vi "changeMode.vi"(8 "error in (no error)":errorcluster, 9 "Mode":T1, 10 "ElectrometerController in":refnum<class "ElectrometerController.lvclass">, 11 "ReadyState in":refnum<class "ReadyState.lvclass">) -> (0 "error out":errorcluster, 2 "ElectrometerController out":refnum<class "ElectrometerController.lvclass">, 3 "ReadyState out":refnum<class "ReadyState.lvclass">)   [LabVIEW 2016, in "ReadyState.lvclass"]
uses:
  ReadyState.lvclass
  ElectrometerController/ElectrometerController.lvclass
  Modes.ctl
  ts_electrometeruserevents/Typedefs/StateValue.ctl
  ts_electrometeruserevents/Typedefs/CommandValue.ctl
  ts_electrometeruserevents/Typedefs/PubDataSV.ctl
  ts_sallv_calibrationelectrometer/DataTypes/logevent_measureType.ctl
  ElectrometerController/ElectrometerController.lvclass/ElectrometerController.ctl
  ts_electrometeruserevents/PubSubDataEvent/PubSubDataEvent.lvclass
  Electrometer.lvclass
  ElectrometerConfiguration/ElectrometerInternalConfiguration.lvclass
  ts_electrometeruserevents/Typedefs/ElectrometerTypedefs.lvlib
  ts_sallv_calibrationelectrometer/SALLV_calibrationElectrometer.lvlib
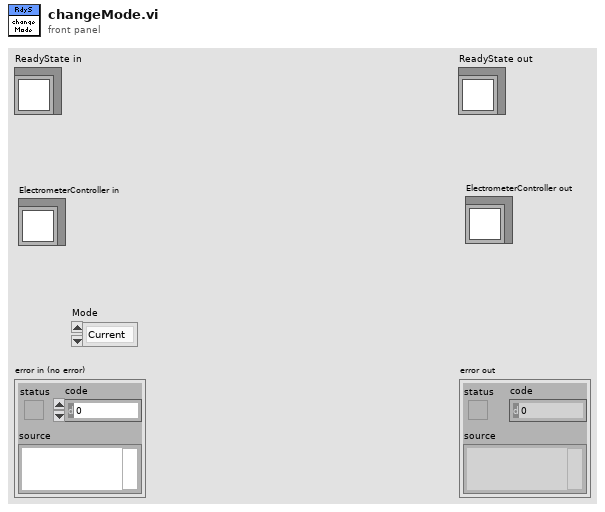
[diagram p1: front panel]
types:
  T1 = typedef "Electrometer.lvclass/Modes.ctl" = enum16{"Current", "Charge"}
  T2 = typedef "SALLV_calibrationElectrometer.lvlib/logevent_measureType.ctl" = cluster{"electId":i16, "mode":u16, "priority":i32}
  T3 = typedef "ElectrometerTypedefs.lvlib/PubDataSV.ctl" = enum16{"DetailedState", "ErrorCode", "Heartbeat", "LoopTime_ms", "LoopTimeOutOfRange", "RejectedCommand", "SummaryState", "Timestamp", "SettingVersions", "SettingsAppliedSerialConfiguration", "AppliedSettingsMatchStart", "InternalState", "Intensity", "MeasureType", "MeasureRange", "DigitalFilterChange", "IntensityReq", "IntegrationTime", "SettingsAppliedReadingSettings"}
  T4 = cluster{"appliedSettingsMatchStart":bool, "Timestamp":dbl}
  T5 = typedef "ElectrometerTypedefs.lvlib/CommandValue.ctl" = enum16{"ClearError", "Disable", "Enable", "Exit", "GoToStandby", "OnHeartbeat", "OnIncomingMessagingError", "OnInterrupt", "Start", "SetDigitalFilter", "StartScan", "StartScanDt", "StartScanReachIntensity", "StopScan", "SetIntegrationTime", "PerformZeroCalib", "SetRange", "SetMode", "Power"}
  T6 = typedef "ElectrometerTypedefs.lvlib/StateValue.ctl" = enum16{"", "DisabledState", "EnabledState", "FaultState", "OffState", "StandbyState", "ReadyState", "ConfiguringState", "ManualReadingState", "UntilIntensityReadingState", "SetDurationReadingState", "BufferReadingState"}
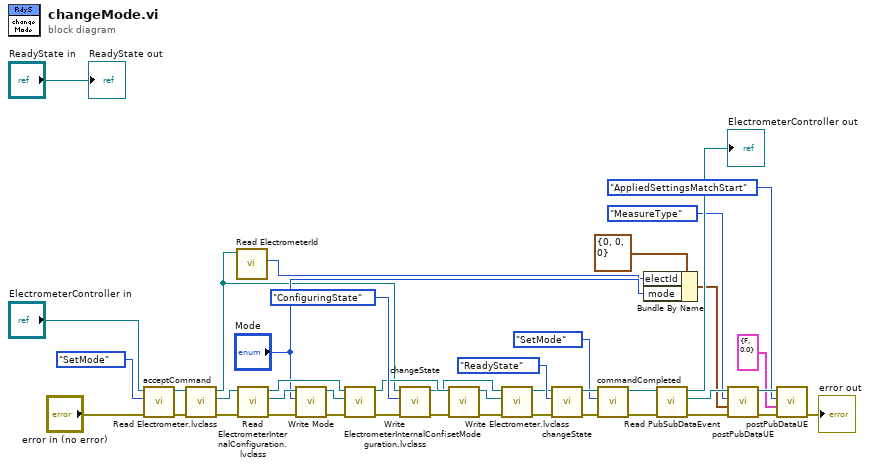
[diagram p0: block diagram]
diagram:
  n1 = call "acceptCommand.vi"("error in (no error)"="error in (no error)", "CommandValue"=CommandValue."SetMode", "ElectrometerController in"="ElectrometerController in") -> ("error out"=w20:errorcluster, "ElectrometerController out"=w21:refnum<class "ElectrometerController.lvclass">)  [unwired: 7 in]
  n2 = call-dynamic "Read Electrometer.lvclass.vi"("error in (no error)"=w20, "ElectrometerController in"=w21) -> ("error out"=w26:errorcluster, "Electrometer.lvclass"=w29:refnum<class "Electrometer.lvclass">, "ElectrometerController out"=w2:refnum<class "ElectrometerController.lvclass">)  [unwired: 7 in]
  n3 = call-dynamic "Read ElectrometerId.vi"("ElectrometerController in"=w2) -> ("ElectrometerId"=w1:enum16{"", "ID1", "ID2"})  [unwired: 8 in, 2 out]
  n4 = call-dynamic "Read ElectrometerInternalConfiguration.lvclass.vi"("error in (no error)"=w26, "Electrometer in"=w29) -> ("error out"=w28:errorcluster, "ElectrometerInternalConfiguration.lvclass"=w32:refnum<class "ElectrometerInternalConfiguration.lvclass">, "Electrometer out"=w30:refnum<class "Electrometer.lvclass">)  [unwired: 7 in]
  n5 = call-dynamic "Write Mode.vi"("error in (no error)"=w28, "Measurement Function (0: Current)"="Mode", "ElectrometerInternalConfiguration in"=w32) -> ("error out"=w27:errorcluster, "ElectrometerInternalConfiguration out"=w31:refnum<class "ElectrometerInternalConfiguration.lvclass">)  [unwired: 7 in]
  n6 = call-dynamic "Write ElectrometerInternalConfiguration.lvclass.vi"("error in (no error)"=w27, "ElectrometerInternalConfiguration.lvclass"=w31, "Electrometer in"=w30) -> ("error out"=w18:errorcluster, "Electrometer out"=w25:refnum<class "Electrometer.lvclass">)  [unwired: 7 in]
  n7 = call "changeState.vi"("error in (no error)"=w18, "StateValue"=StateValue."ConfiguringState", "ElectrometerController in"=w2) -> ("error out"=w41:errorcluster, "ElectrometerController out"=w19:refnum<class "ElectrometerController.lvclass">)  [unwired: 7 in]
  n8 = call "setMode.vi"("error in (no error)"=w41, "Electrometer in"=w25) -> ("error out"=w23:errorcluster, "Electrometer out"=w24:refnum<class "Electrometer.lvclass">)  [unwired: 8 in]
  n9 = call-dynamic "Write Electrometer.lvclass.vi"("error in (no error)"=w23, "Electrometer.lvclass"=w24, "ElectrometerController in"=w19) -> ("error out"=w22:errorcluster, "ElectrometerController out"=w17:refnum<class "ElectrometerController.lvclass">)  [unwired: 7 in]
  n10 = call "changeState.vi"("error in (no error)"=w22, "StateValue"=StateValue."ReadyState", "ElectrometerController in"=w17) -> ("error out"=w34:errorcluster, "ElectrometerController out"=w35:refnum<class "ElectrometerController.lvclass">)  [unwired: 7 in]
  n11 = call "commandCompleted.vi"("error in (no error)"=w34, "CommandValue"=CommandValue."SetMode", "ElectrometerController in"=w35) -> ("error out"=w10:errorcluster, "ElectrometerController out"=w11:refnum<class "ElectrometerController.lvclass">)  [unwired: 7 in]
  n12 = Bundle By Name(cluster=T2 {"electId"=0, "mode"=0, "priority"=0} ("logevent_measureType"), "electId"=w1, "mode"="Mode") -> (w3:T2)
  n13 = call "Read PubSubDataEvent.vi"("error in (no error)"=w10, "ElectrometerController in"=w11) -> ("error out"=w16:errorcluster, "PubSubDataEvent.lvclass"=w15:refnum<class "PubSubDataEvent.lvclass">, "ElectrometerController out"=→"ElectrometerController out":refnum<class "ElectrometerController.lvclass">)  [unwired: 7 in]
  n14 = call "postPubDataUE.vi"("error in (no error)"=w16, "value"=w3, "pubDataSV"=PubDataSV."MeasureType", "PubSubDataEvent in"=w15) -> ("error out"=w14:errorcluster, "PubSubDataEvent out"=w13:refnum<class "PubSubDataEvent.lvclass">)  [unwired: 6 in]
  n15 = call "postPubDataUE.vi"("error in (no error)"=w14, "value"=T4 {"appliedSettingsMatchStart"=FALSE, "Timestamp"=0.0} ("event data"), "pubDataSV"=PubDataSV."AppliedSettingsMatchStart", "PubSubDataEvent in"=w13) -> ("error out"=→"error out":errorcluster)  [unwired: 6 in, 1 out]
  "ReadyState out" <- "ReadyState in"
